vi "Global 1.vi"() -> ()   [LabVIEW 2013]
panel:
  out "disp stop":bool
  out "v2":dbl
  out "v1":dbl
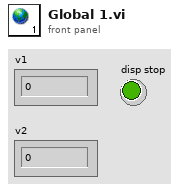
[diagram p1: front panel]
diagram:
